vi "SetThreadValid.vi"(11 "YActor in":refnum<class "YActor.lvclass">) -> (3 "YActor out":refnum<class "YActor.lvclass">)   [LabVIEW 2021, in "YActor.lvclass"]
uses:
  YActor.lvclass
  YActor.lvclass/YActor.ctl
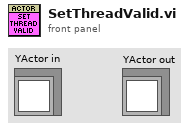
[diagram p1: front panel]
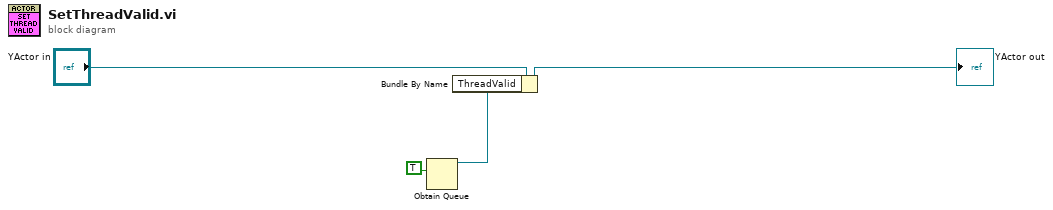
[diagram p0: block diagram]
diagram:
  n1 = Obtain Queue(element data type=TRUE) -> (queue out=w2:refnum<queue>)  [unwired: 4 in, 2 out]
  n2 = Bundle By Name(cluster="YActor in", "ThreadValid"=w2) -> (→"YActor out":refnum<class "YActor.lvclass">)
